vi "F(x,a).vi"(3 "output control":T1, 4 "data":variant, 5 "X":dbl[](array[numeric]), 6 "a":dbl[](array[numeric])) -> (0 "error out":errorcluster, 1 "f'(X,a)":dbl[][](array[numeric]), 2 "f(X,a)":dbl[](array[numeric]))   [LabVIEW 2025]
doc: "This template is the starting point for creating a model function to be passed to the Nonlinear Curve Fit.vi."
uses:
  <vilib>/gmath/NumericalOptimization/LM_output select.ctl
  F(x,a) Cluster.ctl
  <vilib>/Analysis/Matrix/Datatypes/RealMatrix.ctl
  <vilib>/Analysis/Matrix/NI_Matrix.lvlib
  <vilib>/gmath/NI_Gmath.lvlib
panel:
  out "v":dbl
  out "u":dbl
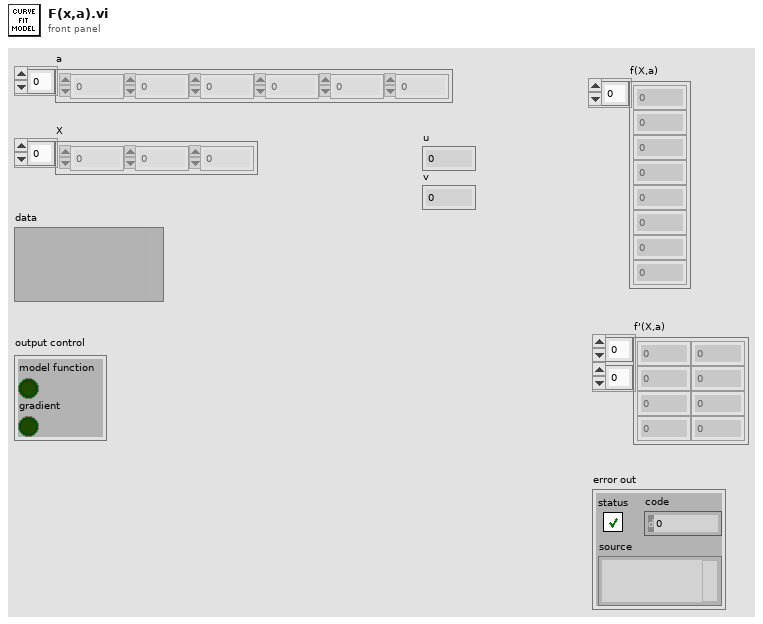
[diagram p1: front panel]
types:
  T1 = typedef "NI_Gmath.lvlib/LM_output select.ctl" = cluster{"model function":bool, "gradient":bool}
  T2 = typedef "F(x,a) Cluster.ctl" = cluster{"R Rotation Matrix":T3, "cx width":dbl, "cy height":dbl, "f_px":dbl, "World corner points (out)":dbl[][]}
  T3 = typedef "NI_Matrix.lvlib/RealMatrix.ctl" = dbl[][]
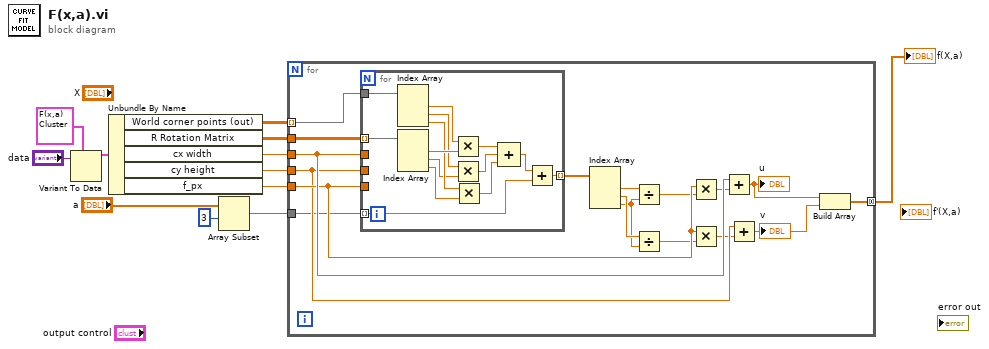
[diagram p0: block diagram]
diagram:
  n1 = Variant To Data(type=T2 {"R Rotation Matrix"=[[0.9588455898290663, 0.17324587630238714, -0.22494666303274574], [-0.11933122759874246, -0.47300100712431575, -0.8729433574861316], [-0.2576338350937756, 0.8638610499400935, -0.43286128657027323]], "cx width"=320.0, "cy height"=240.0, "f_px"=3657.616736883629, "World corner points (out)"=[[-3.25, -3.25, 0.0], [3.25, -3.25, 0.0], [3.25, 3.25, 0.0], [-3.25, 3.25, 0.0]]} ("Cluster"), Variant="data") -> (data=w12:T2)  [unwired: 1 in, 1 out]
  n2 = Unbundle By Name(w12) -> ("World corner points (out)"=w1:dbl[][], "R Rotation Matrix"=w9:T3, "cx width"=w8:dbl, "cy height"=w6:dbl, "f_px"=w7:dbl)
  n3 = Array Subset(array="a", index=3) -> (w3:dbl[])  [unwired: 1 in]
  n4 = for {
    tunnel: w9 -> [w29]
    tunnel: w8 -> [w28]
    tunnel: w7 -> [w27]
    tunnel: w6 -> [w26]
    tunnel: [w25] -> w5 mode=concatenating
    tunnel: w3 -> [w24]
    tunnel: w1 -> [w13] mode=indexing
    n5 = for {
      tunnel: w13 -> [w40]
      tunnel: w29 -> [w43] mode=indexing
      tunnel: w28 -> [_]
      tunnel: w26 -> [_]
      tunnel: w27 -> [_]
      tunnel: [w31] -> w23 mode=indexing
      tunnel: w24 -> [w30] mode=indexing
      n6 = Index Array(array=w40) -> (element #1=w39:dbl, element #2=w38:dbl, element #3=w37:dbl)  [unwired: 3 in]
      n7 = Index Array(array=w43) -> (element #1=w42:dbl, element #2=w36:dbl, element #3=w35:dbl)  [unwired: 3 in]
      n8 = Multiply(x=w39, y=w42) -> (x*y=w41:dbl)
      n9 = Multiply(x=w38, y=w36) -> (x*y=w34:dbl)
      n10 = Multiply(x=w37, y=w35) -> (x*y=w33:dbl)
      n11 = Compound Arithmetic op=ADD(w41, w34, w33) -> (w32:dbl)
      n12 = Add(x=w32, y=w30) -> (x+y=w31:dbl)
    }
    n13 = Index Array(array=w23) -> (element #1=w22:dbl, element #2=w21:dbl, element #3=w20:dbl)  [unwired: 3 in]
    n14 = Divide(x=w22, y=w20) -> (x/y=w19:dbl)
    n15 = Divide(x=w21, y=w20) -> (x/y=w17:dbl)
    n16 = Multiply(x=w27, y=w19) -> (x*y=w18:dbl)
    n17 = Multiply(x=w27, y=w17) -> (x*y=w16:dbl)
    n18 = Add(x=w28, y=w18) -> (x+y=w15:dbl)
    "u" <- w15
    n19 = Add(x=w26, y=w16) -> (x+y=w14:dbl)
    "v" <- w14
    n20 = Build Array(w15, w14) -> (w25:dbl[])
  }
  "f(X,a)" <- w5
